vi "1D Inverse DST.vi"(11 "DST {X}":dbl[](array[numeric])) -> (0 "error":i32, 3 "X":dbl[](array[numeric]))   [LabVIEW 2010, in "NI_AALPro.lvlib"]
doc: "Computes the inverse Discrete Sine Transform (DST) of the input sequence <B>DST {X}</B>. Wire data to the <B>DST {X}</B> input to determine the polymorphic instance to use or manually select the instance."
uses:
  NI_AALPro.lvlib
  lvanlys.dll
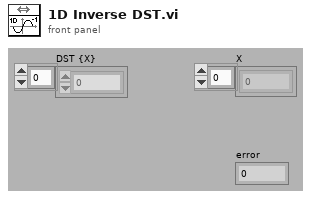
[diagram p1: front panel]
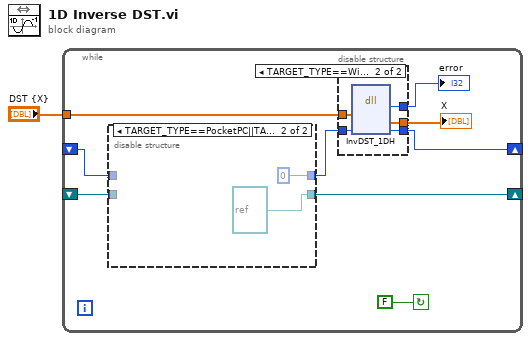
[diagram p0: block diagram]
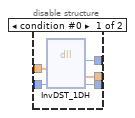
[diagram p2: hidden frame]
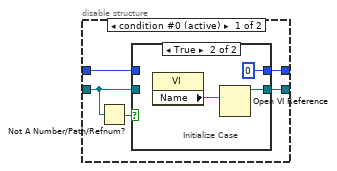
[diagram p3: hidden frame]
diagram:
  n1 = while {
    shift-left: _ -> [w8]
    shift-right: [w3] -> _
    tunnel: "DST {X}" -> [w9]
    shift-right: [w7] -> _
    shift-left: _ -> [w6]
    stop <- FALSE continue-if-true
    n2 = disable-structure shown="TARGET_TYPE==PocketPC||TARGET_TYPE==PalmOS||TARGET_TYPE==FPGA||TARGET_TYPE==Embedded" {
      disable-tunnel: w6 -> [w23 _]
      disable-tunnel: [w24 refnum<vi> refnum ("VI Refnum")] -> w7
      disable-tunnel: w8 -> [w22 _]
      disable-tunnel: [w21 0 ("t")] -> w4
      frame condition #0 (active) {
        n3 = Not A Number/Path/Refnum?(number/path/refnum=w23) -> (NaN/Path/Refnum?=w25:bool)
        n4 = case shown="True" w25 {
          tunnel: [w27 w30] -> w24
          tunnel: w23 -> [w27 _]
          tunnel: w22 -> [w26 _]
          tunnel: [w26 0 ("error")] -> w21
          frame False {
          }
          frame True {
            # "Initialize Case"
            n5 = property class="VI"() -> ("Name"=w28:string)  [unwired: 2 in, 2 out]
            n6 = Open VI Reference(vi path=w28) -> (vi reference=w30:refnum<vi>)  [unwired: 5 in, 1 out]
          }
        }
      }
      frame condition #1 {
      }
    }
    n7 = disable-structure shown="TARGET_TYPE==Windows||TARGET_TYPE==Mac||TARGET_TYPE==Unix" {
      disable-tunnel: w9 -> [w15 w20]
      disable-tunnel: [w14 w19] -> w5
      disable-tunnel: w4 -> [w13 w18]
      disable-tunnel: [w12 w17] -> w3
      disable-tunnel: [w11 w16] -> w2
      frame condition #0 {
        n8 = dll-call lib="C:/Program Files/National Instruments/LabVIEW 2010/resource/lvanlys.*" fn="InvDST_1DH"("xH"=w15, "tbl"=w13) -> (w14:i32, "yH"=w11:dbl[], "tbl"=w12:i32)  [unwired: 5 in, 2 out]
      }
      frame condition #1 (active) {
        n9 = dll-call lib="C:/Program Files/National Instruments/LabVIEW 2010/resource/lvanlys.dll" fn="InvDST_1DH"("xH"=w20, "tbl"=w18) -> ("return type"=w19:i32, "yH"=w16:dbl[], "tbl"=w17:i64)  [unwired: 5 in, 2 out]
      }
    }
    "error" <- w5
    "X" <- w2
  }
